vi "simulacion_control_SISO.vi"() -> ()   [LabVIEW 2017]
uses:
  <vilib>/addons/Control Design/_Model Construction/Data Typedefs.llb/CD Variables.ctl
  <vilib>/Simulation/Scripting/Companion Diagram/SimConfigNode/SimParams.ctl
  <vilib>/Simulation/Scripting/Companion Diagram/SimConfigNode/_simSolvers.ctl
  <vilib>/Simulation/Implementation/Shared/SIMSCR Execution Mode.ctl
  <vilib>/Platform/TimedLoop/XDataNode/timing_clust.ctl
  <vilib>/Platform/TimedLoop/XDataNode/nitl_modes.ctl
  <vilib>/Platform/TimedLoop/XDataNode/wakeup.ctl
  <vilib>/Simulation/Param Hierarchy/Typedefs/SIMPH Param Control Actions.ctl
  <vilib>/Simulation/Implementation/Shared/SIM limit type.ctl
  <vilib>/Simulation/Implementation/Shared/NILVSim_ParamChanged.vi
  <vilib>/Simulation/Implementation/Shared/NILVSim_FinishedLate.vi
  <vilib>/Simulation/Implementation/Shared/NILVSIM_BeginStep.vi
  <vilib>/Simulation/DataSources/Implementation/NILVSim Pulse Generator.llb/SIM Pulse Generator (scalar).vi
  <vilib>/Simulation/Utility/Implementation/SIM Halt.vi
  <vilib>/Simulation/ContinuousLinear/Implementation/NILVSim Integrator new.llb/SIM Integrator distributor (scalar).vi
  <vilib>/Simulation/SignalArithmetic/Implementation/NILVSim Gain.llb/SIM Gain (scalar).vi
  <vilib>/Simulation/ContinuousLinear/Implementation/NILVSim Integrator new.llb/SIM Integrator collector (scalar).vi
  <vilib>/Simulation/ContinuousLinear/Implementation/NILVSim Derivative.llb/SIM derivative (scalar).vi
  <vilib>/Simulation/SignalDisplay/Implementation/NILVSim Time Waveform.llb/SIM Time Waveform (vector).vi
  <vilib>/Simulation/ContinuousLinear/Implementation/NILVSim Transfer Function.llb/SIM Transfer Function Distributor (SISO CD).vi
  <vilib>/Simulation/ContinuousLinear/Implementation/NILVSim Transfer Function.llb/SIM Transfer Function Collector (SISO).vi
  <vilib>/Simulation/Implementation/Shared/NILVSim_Manager.vi
  <vilib>/Utility/error.llb/Clear Errors.vi
  <vilib>/Simulation/Implementation/Shared/NILVSim_FinalizeModel.vi
  <vilib>/addons/Control Design/_Model Construction/Model Creation.llb/Model Creation SubVI/cd_Create Symbolic Transfer Function Model.vi
  <vilib>/addons/Control Design/_Utility/Model Viewer.llb/Model Viewer SubVI/cd_Draw Transfer Function Equation (TF).vi
  <vilib>/picture/3D Picture Control/Object/Create Object (drawable).vi
  <vilib>/Simulation/Implementation/Shared/SIM Unbundle Sim Info.vi
  <vilib>/Simulation/Implementation/Shared/SIMSH Read Queue.vi
  <vilib>/Simulation/Implementation/Shared/NILVSim_Initialize.vi
  <vilib>/picture/3D Picture Control/Transformations/Rotate Z-axis.vi
  <vilib>/picture/3D Picture Control/Object/Add Object.vi
  <vilib>/picture/3D Picture Control/Object/Add Object (reference).vi
  <vilib>/Simulation/Utility/Implementation/NILVSim Get Time and IsAcceptedStep.vi
  <vilib>/Simulation/Implementation/Shared/NILVSim_GetModelError.vi
  <vilib>/Simulation/Implementation/Shared/SIM Bundle Sim Info.vi
  <vilib>/Simulation/Scripting/Companion Diagram/SimConfigNode/SimDog.xnode
  <vilib>/Platform/TimedLoop/XDataNode/XDataNode.xnode
  <vilib>/Simulation/Implementation/XNodeFramework/SimXNode/SimX.xnode
  <vilib>/addons/Control Design/_Model Construction/NI_LinSys_Model Creation.lvlib
  <vilib>/addons/Control Design/_Utility/NI_CD_Model Viewer.lvlib
  <vilib>/addons/Control Design/_Model Construction/Model Typedefs.llb/CD General Elements.ctl
  <vilib>/addons/Control Design/_Model Construction/NI_LinSys_Model Typedefs.lvlib
  <vilib>/addons/Control Design/_Model Construction/Model Typedefs.llb/CD Transfer Function Model (SISO).ctl
  <vilib>/addons/Control Design/_Model Construction/Model Typedefs.llb/CD Transfer Function Model (MIMO).ctl
  <vilib>/Simulation/ContinuousLinear/Implementation/NILVSim Integrator new.llb/SIM Integrator (scalar).vi
  <vilib>/Simulation/ContinuousLinear/Implementation/NILVSim Transfer Function.llb/SIM Transfer Function (SISO CD).vi
  <vilib>/picture/3D Picture Control/NI_3D Picture Control.lvlib
  <vilib>/Platform/TimedLoop/XDataNode/XDNodeRunTimeDep.lvlib
  <vilib>/Simulation/Implementation/Shared/NI_SIM_Implementation.lvlib
  <vilib>/addons/Control Design/_Model Construction/NI_LinSys_Data Typedefs.lvlib
panel:
  out "3D Picture":refnum<vi>(3d-picture)
  in  "Kd 2":dbl=1.0
  in  "Ki 2":dbl=0.05
  in  "Kp":dbl=5.0
  in  "Halt?":bool
  in  "Selector":bool
  out "Waveform Chart":waveform(dbl)[](graph)=[{"t0"=timestamp(10 s since 1904-01-01), "dt"=1.0, "Y"=[3.14]}, {"t0"=timestamp(10 s since 1904-01-01), "dt"=1.0, "Y"=[1.627249712833804e+306]}]
  out "P":dbl(knob)=1.627249712833804e+306 scale=-3.14..3.14
  in  "SP":dbl(knob)=2.220357231105655 scale=-3.14..3.14
  out "Equation":picture
  in  "Variables":T1=[{"Name"="Km", " Value"=0.028}, {"Name"="Jeq", " Value"=3.3}, {"Name"="Rm", " Value"=9.64e-06}] {"Value" format="%.2g"}
  in  "Symbolic Denominator":string[](array[string])=["Km^2", "Jeq*Rm"]
  in  "Symbolic Numerator":string[](array[string])=["Km"]
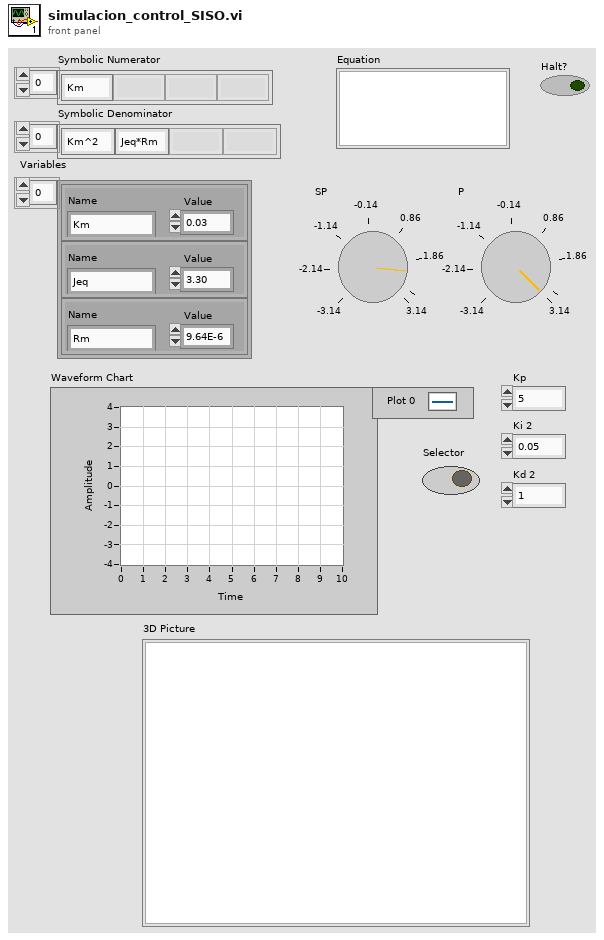
[diagram p1: front panel]
types:
  T1 = typedef "NI_LinSys_Data Typedefs.lvlib/CD Variables.ctl" = cluster{"Name":string, " Value":dbl}[]
  T2 = cluster{"Red":sgl, "Green":sgl, "Blue":sgl, "Alpha":sgl}
  T3 = typedef "NI_LinSys_Model Typedefs.lvlib/CD Transfer Function Model (MIMO).ctl" = cluster{"properties":T4, "transfer function(s)":T5[][]}
  T4 = typedef "NI_LinSys_Model Typedefs.lvlib/CD General Elements.ctl" = cluster{"Model name":string, "Input names":string[], "Output names":string[], "Input Delays":dbl[], "Output Delays":dbl[], "Sampling Time":dbl, "Notes":string}
  T5 = typedef "NI_LinSys_Model Typedefs.lvlib/CD Transfer Function Model (SISO).ctl" = cluster{"Numerator":dbl[], "Denominator":dbl[], "delay":dbl}
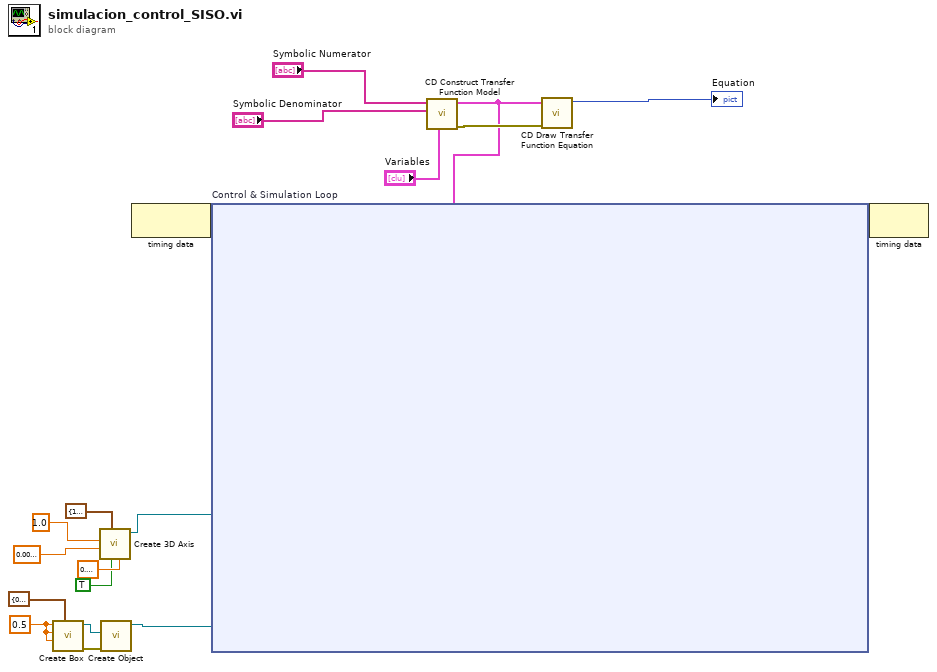
[diagram p0: block diagram]
diagram:
  w11 = sgl 0.5 ("Length X")
  n1 = call <vilib>:"Create Box.vi"("Color"=T2 {"Red"=0.0, "Green"=1.0, "Blue"=0.0, "Alpha"=1.0}, "Length Z"=w11, "Length Y"=w11, "Length X"=w11) -> ("error out"=w9:errorcluster, "New Box Refnum"=w8:refnum<vi>)  [unwired: 6 in]
  n2 = call <vilib>:"Create 3D Axis.vi"("Character Size"=sgl 0.1, "Axis label?"=TRUE, "Color"=T2 {"Red"=1.0, "Green"=0.0, "Blue"=0.0, "Alpha"=1.0}, "Radius"=sgl 0.01, "Length"=sgl 1.0) -> ("New Object Refnum"=w2:refnum<vi>)  [unwired: 5 in, 1 out]
  n3 = call-poly <vilib>:"Create Object.vi"("error in (no error)"=w9, "Geometry"=w8) -> ("Scene:New Object"=w1:refnum<vi>)  [unwired: 8 in, 1 out]
  n4 = node-c288() -> (w14:variant)  [unwired: 1 in]
  n5 = call-poly <vilib>:"CD Construct Transfer Function Model.vi"("Variables"="Variables", "Symbolic Denominator"="Symbolic Denominator", "Symbolic Numerator"="Symbolic Numerator") -> ("error out"=w16:errorcluster, "Transfer Function Model"=w12:T3)  [unwired: 7 in]
  n6 = node-c254 "Control & Simulation Loop"(w14, w12, w2, w1) -> (w13:variant)
  n7 = call-poly <vilib>:"CD Draw Transfer Function Equation.vi"("error in (no error)"=w16, "Transfer Function Model"=w12) -> ("Equation"=→"Equation":picture)  [unwired: 7 in, 2 out]
  n8 = node-c288(w13) -> ()  [unwired: 1 out]
